vi "Close.vi"(8 "error in (no error)":errorcluster, 11 "1553 Component in":refnum<class "1553 Component.lvclass">) -> (0 "error out":errorcluster)   [LabVIEW 2020, in "BCI-1553 API.lvlib" / "1553 Component.lvclass"]
doc: "Closes all the resources allocated by this component. It is strongly suggested to call the 'Clean Up' method before closing a component."
uses:
  1553 Component.lvclass
  1553 Component.lvclass/1553 Component.ctl
  Dependencies/FPGA Interface/FPGA Interface.lvclass
  Dependencies/Virtual Memory Unit/Virtual Memory Unit.lvclass
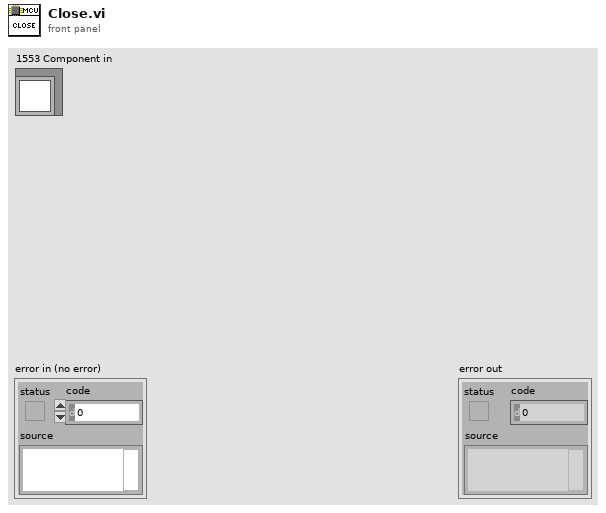
[diagram p1: front panel]
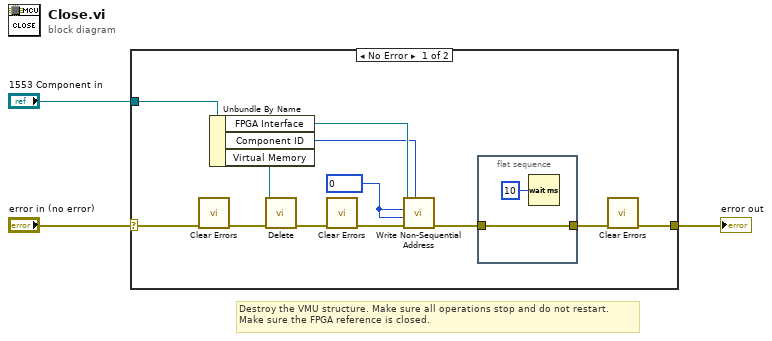
[diagram p0: block diagram]
diagram:
  # "Destroy the VMU structure. Make sure all operations stop and do not restart.\nMake sure the FPGA reference is closed."
  n1 = case shown="No Error" "error in (no error)" {
    selector: "error in (no error)" -> [w12 w18]
    tunnel: [w11 w18] -> w2
    tunnel: "1553 Component in" -> [w15 _]
    frame No Error {
      w6 = u16 0 ("Address")
      n2 = call <vilib>:"Clear Errors.vi"("error in (no error)"=w12) -> ("error out"=w10:errorcluster)  [unwired: 5 in, 1 out]
      n3 = Unbundle By Name(w15) -> ("FPGA Interface"=w8:refnum<class "FPGA Interface.lvclass">, "Component ID"=w7:u8, "Virtual Memory"=w13:refnum<class "Virtual Memory Unit.lvclass">)
      n4 = call "Delete.vi"("error in (no error)"=w10, "Virtual Memory Unit in"=w13) -> ("error out"=w14:errorcluster)  [unwired: 9 in]
      n5 = call <vilib>:"Clear Errors.vi"("error in (no error)"=w14) -> ("error out"=w9:errorcluster)  [unwired: 5 in, 1 out]
      n6 = call-dynamic "Write Non-Sequential Address.vi"("Target IC (1-8)"=w7, "error in (no error)"=w9, "Data"=w6, "Address"=w6, "FPGA Interface in"=w8) -> ("error out"=w5:errorcluster)  [unwired: 6 in]
      n7 = flat-sequence {
        tunnel: [w17] -> w4
        tunnel: w5 -> [w17]
        frame #0 {
          n8 = Wait (ms)(milliseconds to wait=u32 10) -> ()  [unwired: 1 out]
        }
      }
      n9 = call <vilib>:"Clear Errors.vi"("error in (no error)"=w4) -> ("error out"=w11:errorcluster)  [unwired: 5 in, 1 out]
    }
    frame Error {
    }
  }
  "error out" <- w2
